vi "myRIO_BRig_RT__Case_Exp_State_initTrial_dataTrial.vi"(8 "input_spout":enum16{"Left", "Right"}(ring), 9 "input_dataCurrent":u16[](array[numeric]), 10 "input_dataExp":u16[](array[numeric]), 11 "input_dataTrial":u16[][](array[numeric])) -> (0 "output_laserPower_l2":u16, 2 "output_dataCurrent":u16[](array[numeric]), 3 "output_dataTrial":u16[][](array[numeric]), 5 "output_laserPower_l1":u16)   [LabVIEW 2014]
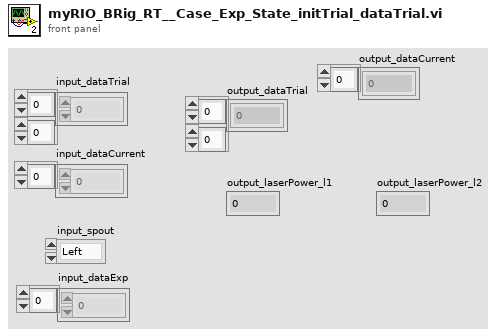
[diagram p1: front panel]
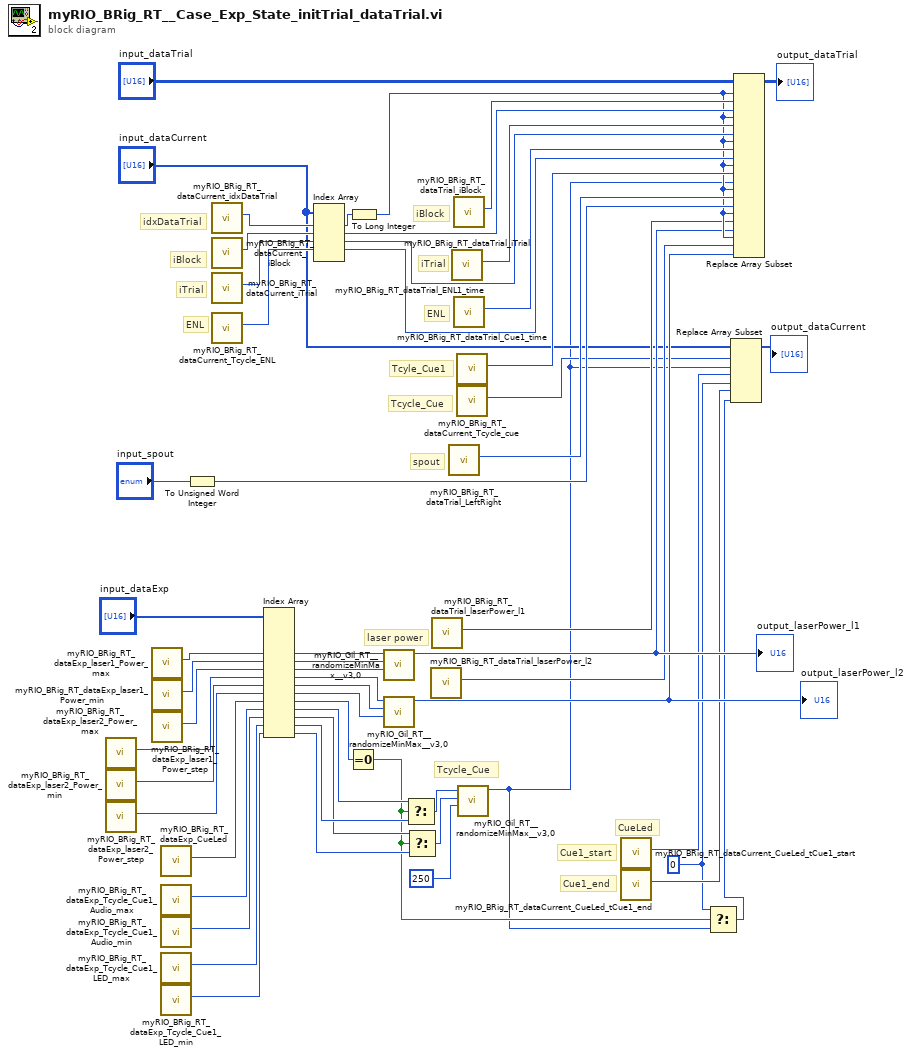
[diagram p0: block diagram]
diagram:
  w2 = u16 0 ("new element/subarray")
  # "Cue1_end"
  # "Cue1_start"
  # "CueLed"
  # "Tcycle_Cue"
  # "laser power"
  # "Tcyle_Cue1"
  # "Tcycle_Cue"
  # "ENL"
  # "ENL"
  # "spout"
  # "iBlock"
  # "iTrial"
  # "idxDataTrial"
  # "iBlock"
  # "iTrial"
  n1 = call "myRIO_BRig_RT_dataExp_laser2_Power_max.vi"() -> ("output_laser2_Power_max"=w33:i32)  [unwired: 11 in]
  n2 = call "myRIO_BRig_RT_dataExp_laser2_Power_min.vi"() -> ("output_laser2_Power_min"=w32:i32)  [unwired: 11 in]
  n3 = call "myRIO_BRig_RT_dataExp_laser2_Power_step.vi"() -> ("output_laser2_Power_step"=w31:i32)  [unwired: 11 in]
  n4 = call "myRIO_BRig_RT_dataExp_laser1_Power_max.vi"() -> ("output_laser1_Power_max"=w39:i32)  [unwired: 11 in]
  n5 = call "myRIO_BRig_RT_dataExp_laser1_Power_min.vi"() -> ("output_laser1_Power_min"=w38:i32)  [unwired: 11 in]
  n6 = call "myRIO_BRig_RT_dataExp_laser1_Power_step.vi"() -> ("output_laser1_Power_step"=w37:i32)  [unwired: 11 in]
  n7 = call "myRIO_BRig_RT_dataExp_CueLed.vi"() -> ("output_CueLed"=w7:i32)  [unwired: 11 in]
  n8 = call "myRIO_BRig_RT_dataExp_Tcycle_Cue1_Audio_max.vi"() -> ("output_Tcycle_Cue1_Audio_max"=w22:i32)  [unwired: 11 in]
  n9 = call "myRIO_BRig_RT_dataExp_Tcycle_Cue1_Audio_min.vi"() -> ("output_Tcycle_Cue1_Audio_min"=w21:i32)  [unwired: 11 in]
  n10 = call "myRIO_BRig_RT_dataExp_Tcycle_Cue1_LED_max.vi"() -> ("output_Tcycle_Cue1_LED_max"=w20:i32)  [unwired: 11 in]
  n11 = call "myRIO_BRig_RT_dataExp_Tcycle_Cue1_LED_min.vi"() -> ("output_Tcycle_Cue1_LED_min"=w19:i32)  [unwired: 11 in]
  n12 = To Unsigned Word Integer(number="input_spout") -> (unsigned 16bit integer=w42:u16)
  n13 = call "myRIO_BRig_RT_dataCurrent_idxDataTrial.vi"() -> ("output_idxDataTrial"=w55:i32)  [unwired: 11 in]
  n14 = call "myRIO_BRig_RT_dataCurrent_iBlock.vi"() -> ("output_iBlock"=w56:i32)  [unwired: 11 in]
  n15 = call "myRIO_BRig_RT_dataCurrent_iTrial.vi"() -> ("output_iTrial"=w57:i32)  [unwired: 11 in]
  n16 = call "myRIO_BRig_RT_dataCurrent_Tcycle_ENL.vi"() -> ("output_ENL"=w46:i32)  [unwired: 11 in]
  n17 = Index Array(array="input_dataExp", index #4=w39, index #5=w38, index #6=w37, index #7=w33, index #8=w32, index #9=w31, index #10=w7, index #11=w22, index #12=w21, index #13=w20, index #14=w19) -> (element #4=w36:u16, element #5=w35:u16, element #6=w34:u16, element #7=w30:u16, element #8=w29:u16, element #9=w28:u16, element #10=w18:u16, element #11=w17:u16, element #12=w15:u16, element #13=w16:u16, element #14=w14:u16)  [unwired: 3 in, 3 out]
  n18 = Index Array(array="input_dataCurrent", index #1=w55, index #2=w56, index #3=w57, index #4=w46) -> (element #1=w54:u16, element #2=w51:u16, element #3=w48:u16, element #4=w44:u16)  [unwired: 1 in, 1 out]
  n19 = Equal To 0?(x=w18) -> (x = 0?=w4:bool)
  n20 = To Long Integer(number=w54) -> (32bit integer=w27:i32)
  n21 = call "myRIO_Gil_RT__randomizeMinMax__v3,0.vi"("Input_Increment"=w34, "Input_Min"=w35, "Input_Max"=w36) -> ("Output"=w25:u16)  [unwired: 8 in]
  "output_laserPower_l1" <- w25
  n22 = call "myRIO_Gil_RT__randomizeMinMax__v3,0.vi"("Input_Increment"=w28, "Input_Min"=w29, "Input_Max"=w30) -> ("Output"=w23:u16)  [unwired: 8 in]
  "output_laserPower_l2" <- w23
  n23 = Select(t=w17, s=w4, f=w16) -> (s? t:f=w13:u16)
  n24 = Select(t=w15, s=w4, f=w14) -> (s? t:f=w12:u16)
  n25 = call "myRIO_BRig_RT_dataTrial_laserPower_l2.vi"() -> ("output_laserPower_l2"=w24:i32)  [unwired: 11 in]
  n26 = call "myRIO_BRig_RT_dataTrial_laserPower_l1.vi"() -> ("output_laserPower_l1"=w26:i32)  [unwired: 11 in]
  n27 = call "myRIO_BRig_RT_dataTrial_LeftRight.vi"() -> ("output_LeftRight"=w43:i32)  [unwired: 11 in]
  n28 = call "myRIO_BRig_RT_dataTrial_iTrial.vi"() -> ("output_iTrial"=w49:i32)  [unwired: 11 in]
  n29 = call "myRIO_BRig_RT_dataTrial_iBlock.vi"() -> ("output_iBlock"=w50:i32)  [unwired: 11 in]
  n30 = call "myRIO_BRig_RT_dataTrial_ENL1_time.vi"() -> ("output_ENL1_time"=w45:i32)  [unwired: 11 in]
  n31 = call "myRIO_BRig_RT_dataTrial_Cue1_time.vi"() -> ("output_Cue1_time"=w41:i32)  [unwired: 11 in]
  n32 = call "myRIO_BRig_RT_dataCurrent_Tcycle_cue.vi"() -> ("output_Tcycle_cue"=w9:i32)  [unwired: 11 in]
  n33 = call "myRIO_Gil_RT__randomizeMinMax__v3,0.vi"("Input_Increment"=u16 250, "Input_Min"=w12, "Input_Max"=w13) -> ("Output"=w1:u16)  [unwired: 8 in]
  n34 = call "myRIO_BRig_RT_dataCurrent_CueLed_tCue1_start.vi"() -> ("output_CueLed_tCue1_start"=w6:i32)  [unwired: 11 in]
  n35 = call "myRIO_BRig_RT_dataCurrent_CueLed_tCue1_end.vi"() -> ("output_CueLed_tCue1_end"=w5:i32)  [unwired: 11 in]
  n36 = Select(t=w2, s=w4, f=w1) -> (s? t:f=w3:u16)
  n37 = Replace Array Subset(array="input_dataCurrent", new element #1=w1, index #1=w9, new element #2=w2, index #2=w6, new element #3=w3, index #3=w5) -> (→"output_dataCurrent":u16[])
  n38 = Replace Array Subset(array="input_dataTrial", new element #1=w51, index (row) #1=w27, index (col) #1=w50, new element #2=w48, index (row) #2=w27, index (col) #2=w49, new element #3=w44, index (row) #3=w27, index (col) #3=w45, new element #4=w1, index (row) #4=w27, index (col) #4=w41, new element #5=w42, index (row) #5=w27, index (col) #5=w43, new element #6=w25, index (row) #6=w27, index (col) #6=w26, new element #7=w23, index (row) #7=w27, index (col) #7=w24) -> (→"output_dataTrial":u16[][])
